vi "msg.next_lua.vi"(5 "LuaVIEW reference":T1) -> (15 "error out":errorcluster)   [LabVIEW 2012]
doc: "Returns the next message and removes it from the task's message queue. The message returned is the oldest message present in the queue. Typically, this function is used when a task must process messages in first-in first-out order after being woken up. Note that multiple messages may be present in the queue, so do not go back to sleep until all have been handled.\nResults:\nany:message, message string or nil when the queue is empty.\nErrors:\nFunction must be called from a task context but was not."
uses:
  typedefs/t_LuaVIEW Reference.ctl
  typedefs/t_LuaVIEW Task State Methods.ctl
  subvis/private/LuaVIEW Push (string).vi
  subvis/private/LuaVIEW Push (nil).vi
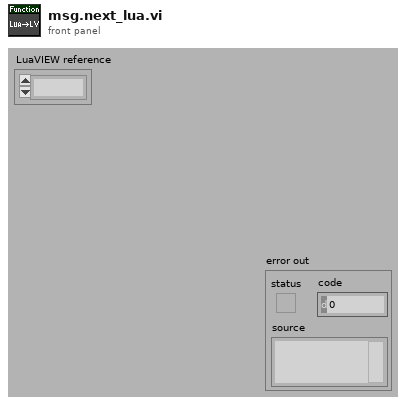
[diagram p1: front panel]
types:
  T1 = typedef "t_LuaVIEW Reference.ctl" = refnum<k1>
  T2 = typedef "t_LuaVIEW Task State Methods.ctl" = enum16{"cleanup", "set initial", "set mode", "set active mode", "set error", "get task info", "get script info", "set signal", "clear signal", "test handled", "test delegated", "test signal", "handle signal", "delegate signal", "allow signal", "disallow signal", "disallow all", "signals?", "delegated signals?", "protection++", "protection--", "protection=0", "message", "next message", "pop message", "message available?", "force stop", "set swap preps", "apply swap preps"}
  T3 = typedef "t_LuaVIEW Task State Pane.ctl" = refnum<vi>
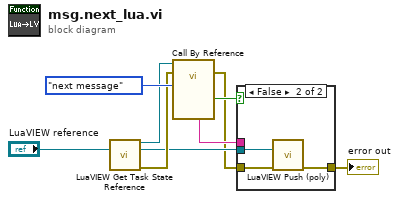
[diagram p0: block diagram]
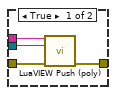
[diagram p2: hidden frame]
diagram:
  n1 = call "LuaVIEW Get Task State Reference.vi"("LuaVIEW reference in"="LuaVIEW reference") -> ("task state reference"=w6:T3, "LuaVIEW reference out"=w3:T1, "error out"=w4:errorcluster)  [unwired: 12 in]
  n2 = call-by-ref "?"(reference=w6, error in=w4, "method"=t_LuaVIEW_Task_State_Methods."next message") -> (error out=w1:errorcluster, "set/available/pending"=w8:bool, "string out"=w7:string)  [unwired: 10 in, 4 out]
  n3 = case shown="False" w8 {
    tunnel: w3 -> [w13 w16]
    tunnel: w7 -> [w12 _]
    tunnel: [w11 w15] -> w2
    tunnel: w1 -> [w10 w14]
    frame True {
      n4 = call-poly "LuaVIEW Push (poly).vi"("string"=w12, "LuaVIEW reference in"=w13, "error in (no error)"=w10) -> ("error out"=w11:errorcluster)  [unwired: 11 in, 1 out]
    }
    frame False {
      n5 = call-poly "LuaVIEW Push (poly).vi"("LuaVIEW reference in"=w16, "error in (no error)"=w14) -> ("error out"=w15:errorcluster)  [unwired: 12 in, 1 out]
    }
  }
  "error out" <- w2
